vi "Triggered Tasks-Stop and Clear.vi"() -> (0 "error out":errorcluster)   [LabVIEW 2013]
uses:
  Globals/gl_Triggering globals.vi
  Pockels/Globals/gl_Pockels control globals.vi
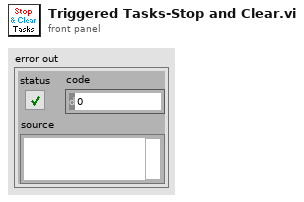
[diagram p1: front panel]
types:
  T1 = typedef "Triggered tasks cluster.ctl" = cluster{"DO task-Encoder trigger":refnum<k21>, "AO Task-Pockels modulation":refnum<k21>, "Counter Clock Task":refnum<k21>}
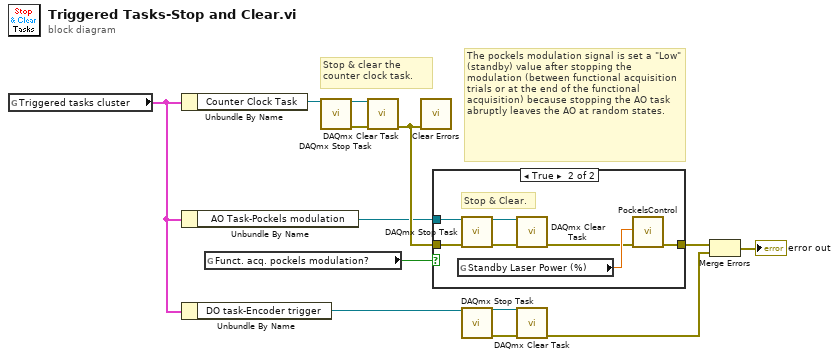
[diagram p0: block diagram]
diagram:
  # "The pockels modulation signal is set a \"Low\" (standby) value after stopping the modulation (between functional acquisition trials or at the end of the functional acquisition) because stopping the AO task abruptly leaves the AO at random states."
  # "Stop & clear the counter clock task."
  n1 = global read "gl_Triggering globals.vi" "Triggered tasks cluster"() -> (w5:T1)
  n2 = Unbundle By Name(w5) -> ("Counter Clock Task"=w8:refnum<k21>)
  n3 = Unbundle By Name(w5) -> ("AO Task-Pockels modulation"=w6:refnum<k21>)
  n4 = Unbundle By Name(w5) -> ("DO task-Encoder trigger"=w9:refnum<k21>)
  n5 = global read "gl_Pockels control globals.vi" "Funct. acq. pockels modulation?"() -> (w7:bool)
  n6 = call <vilib>:"DAQmx Stop Task.vi"("task/channels in"=w8) -> ("task out"=w4:refnum<k21>, "error out"=w3:errorcluster)  [unwired: 13 in]
  n7 = call <vilib>:"DAQmx Clear Task.vi"("task in"=w4, "error in"=w3) -> ("error out"=w11:errorcluster)  [unwired: 13 in]
  n8 = call <vilib>:"Clear Errors.vi"("error in (no error)"=w11) -> ()  [unwired: 6 in, 1 out]
  n9 = case shown="True" w7 {
    tunnel: [w14 w15] -> w10
    tunnel: w6 -> [_ w19]
    tunnel: w11 -> [w14 w18]
    frame False {
    }
    frame True {
      # "Stop & Clear."
      n10 = global read "gl_Pockels control globals.vi" "Standby Laser Power (%)"() -> (w17:dbl)
      n11 = call <vilib>:"DAQmx Stop Task.vi"("task/channels in"=w19, "error in"=w18) -> ("task out"=w21:refnum<k21>, "error out"=w20:errorcluster)  [unwired: 12 in]
      n12 = call <vilib>:"DAQmx Clear Task.vi"("task in"=w21, "error in"=w20) -> ("error out"=w16:errorcluster)  [unwired: 13 in]
      n13 = call "PockelsControl.vi"("Error In"=w16, "Laser Power (%)"=w17) -> ("Error Out"=w15:errorcluster)  [unwired: 9 in]
    }
  }
  n14 = call <vilib>:"DAQmx Stop Task.vi"("task/channels in"=w9) -> ("task out"=w2:refnum<k21>, "error out"=w12:errorcluster)  [unwired: 13 in]
  n15 = call <vilib>:"DAQmx Clear Task.vi"("task in"=w2, "error in"=w12) -> ("error out"=w13:errorcluster)  [unwired: 13 in]
  n16 = Merge Errors(w10, w13) -> (→"error out":errorcluster)
